vi "add code verifier to URI.vi"(8 "error in (no error)":errorcluster, 10 "URI in":refnum<class "URI.lvclass">, 11 "Oauth2 in":refnum<class "Oauth2.lvclass">) -> (0 "error out":errorcluster, 2 "URI out":refnum<class "URI.lvclass">, 3 "Oauth2 out":refnum<class "Oauth2.lvclass">)   [LabVIEW 2017, in "Oauth2.lvclass"]
uses:
  Oauth2.lvclass
  <vilib>/LabVIEW Open Source Project/OpenURI/uri/URI.lvclass
  Oauth2.lvclass/Oauth2.ctl
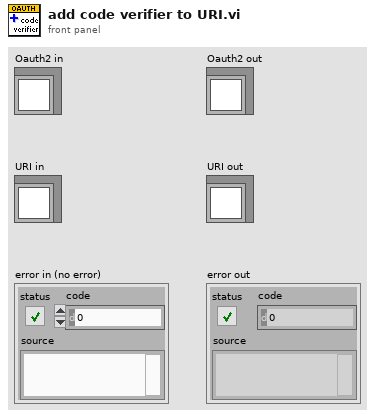
[diagram p1: front panel]
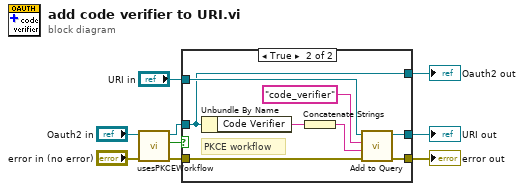
[diagram p0: block diagram]
diagram:
  n1 = call "usesPKCEWorkflow.vi"("error in (no error)"="error in (no error)", "Oauth2 in"="Oauth2 in") -> ("error out"=w6:errorcluster, "PKCE?"=w7:bool, "Oauth2 out"=w8:refnum<class "Oauth2.lvclass">)  [unwired: 7 in]
  n2 = case shown="True" w7 {
    tunnel: "URI in" -> [w11 w20]
    tunnel: [w11 w19] -> w2
    tunnel: w6 -> [w12 w18]
    tunnel: [w12 w17] -> w3
    tunnel: w8 -> [w10 w15]
    tunnel: [w10 w15] -> w9
    frame False {
    }
    frame True {
      # "PKCE workflow"
      n3 = Unbundle By Name(w15) -> ("Code Verifier"=w14:string)
      n4 = Concatenate Strings(w14) -> (w13:string)
      n5 = call <vilib>:"Add to Query.vi"("error in (no error)"=w18, "value"=w13, "key"="code_verifier", "URI in"=w20) -> ("error out"=w17:errorcluster, "URI out"=w19:refnum<class "URI.lvclass">)  [unwired: 6 in]
    }
  }
  "Oauth2 out" <- w9
  "error out" <- w3
  "URI out" <- w2
